vi "Total Time.vi"() -> ()   [LabVIEW 2013]
panel:
  in  "Total Time":dbl
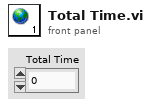
[diagram p1: front panel]
diagram:
